vi "Query Files.vi"(8 "error in (no error)":errorcluster, 11 "NI Skyline Configuration HTTP in":refnum<class "NI Skyline Configuration HTTP.lvclass">) -> (0 "error out":errorcluster, 2 "file ids":string[](array[string]), 3 "NI Skyline Configuration HTTP out":refnum<class "NI Skyline Configuration HTTP.lvclass">)   [LabVIEW 2019]
uses:
  <vilib>/Skyline/Configuration/Configuration HTTP_class/NI Skyline Configuration HTTP.lvclass
  <vilib>/Skyline/Configuration/Configuration HTTP_class/NI Skyline Configuration HTTP.lvclass/NI Skyline Configuration HTTP.ctl
  <vilib>/Skyline/Configuration/Configuration HTTP_class/Read Server URL.vi
  <vilib>/httpClient/POSTBuffer.vi
  <vilib>/httpClient/LabVIEWHTTPClient.lvlib
panel:
  in  "take":i32
  in  "skip":i32
  out "total file count":i32
  out "files returned":i32
  out "body":string
  out "url":string
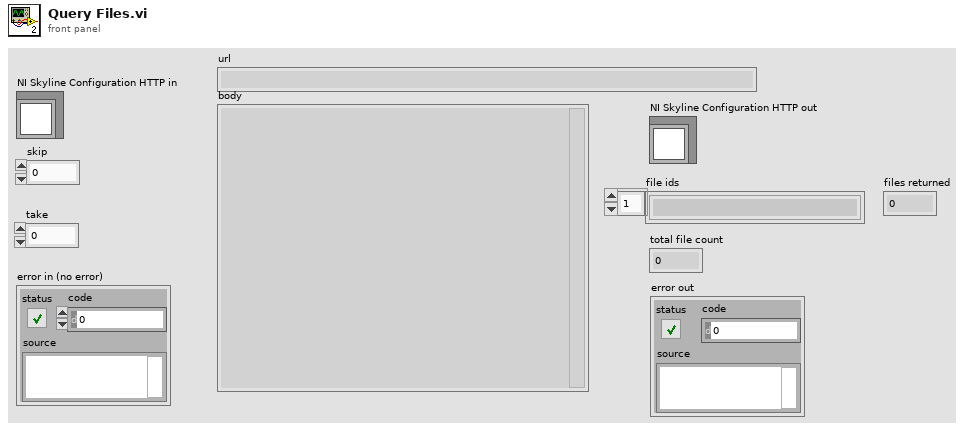
[diagram p1: front panel]
types:
  T1 = typedef "LabVIEWHTTPClient.lvlib/ClientHandle.ctl" = refnum<k1>
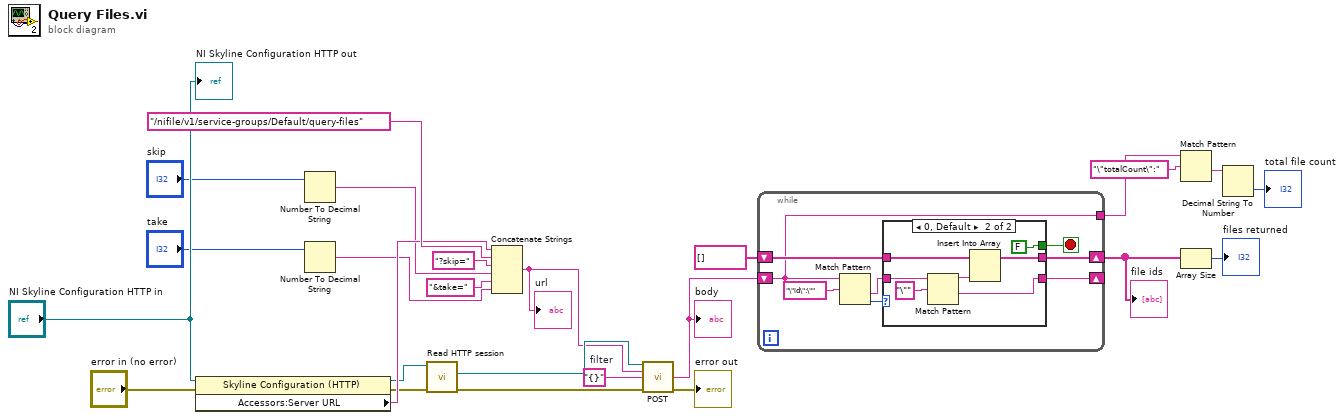
[diagram p0: block diagram]
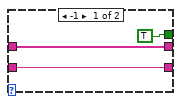
[diagram p2: hidden frame]
diagram:
  w15 = "{}"  # filter
  n1 = property class="Skyline Configuration (HTTP)"(reference="NI Skyline Configuration HTTP in", error in="error in (no error)") -> (reference out=w22:refnum<class "NI Skyline Configuration HTTP.lvclass">, error out=w23:errorcluster, "Accessors:Server URL"=w24:string)
  n2 = Number To Decimal String(number="skip") -> (decimal integer string=w3:string)  [unwired: 1 in]
  n3 = Number To Decimal String(number="take") -> (decimal integer string=w1:string)  [unwired: 1 in]
  n4 = call <vilib>:"Read HTTP session.vi"("error in (no error)"=w23, "HTTP configuration in"=w22) -> ("error out"=w14:errorcluster, "http session"=w17:T1)  [unwired: 7 in, 1 out]
  n5 = Concatenate Strings(w24, "/nifile/v1/service-groups/Default/query-files" ("string"), "?skip=" ("string"), w3, "&take=" ("string"), w1) -> (w16:string)
  "url" <- w16
  n6 = call-poly <vilib>:"POST.vi"("client handle"=w17, "url"=w16, "buffer"=w15, "error in (no error)"=w14) -> ("body"=w12:string, "error out"=→"error out":errorcluster)  [unwired: 8 in, 2 out]
  "body" <- w12
  n7 = while {
    shift-right: [w29] -> _
    shift-left: w12 -> [w26]
    shift-right: [w28] -> w11
    shift-left: string[] [] -> [w27]
    tunnel: [w26] -> w7
    stop <- w30 stop-if-true
    n8 = Match Pattern(string=w26, regular expression="\"id\":\"") -> (after substring=w32:string, offset past match=w31:i32)  [unwired: 1 in, 2 out]
    n9 = case shown="0, Default" w31 {
      tunnel: w32 -> [w34 w43]
      tunnel: [TRUE FALSE] -> w30
      tunnel: [w34 w40] -> w29
      tunnel: [w35 w38] -> w28
      tunnel: w27 -> [w35 w37]
      frame -1 {
      }
      frame 0, Default {
        n10 = Match Pattern(string=w43, regular expression="\"") -> (before substring=w39:string, after substring=w40:string)  [unwired: 1 in, 2 out]
        n11 = Insert Into Array(array=w37, new element=w39) -> (w38:string[])  [unwired: 1 in]
      }
    }
  }
  "file ids" <- w11
  n12 = Match Pattern(string=w7, regular expression="\"totalCount\":") -> (after substring=w5:string)  [unwired: 1 in, 3 out]
  n13 = Array Size(array=w11) -> (size(s)=→"files returned":i32)
  n14 = Decimal String To Number(string=w5) -> (number=→"total file count":i32)  [unwired: 2 in, 1 out]
  "NI Skyline Configuration HTTP out" <- "NI Skyline Configuration HTTP in"
